vi "Graph.vi"(5 "Caption.Text":string="Frequency Responce UUT", 6 "Y Scale.Name Label.Text":string="Level/dBSPL", 7 "X Scale.Name Label.Text":string="Frequency/Hz", 9 "LimitHigh":cluster{"x-Axis":dbl[], "y-Axis":dbl[]}={"x-Axis"=[0.0, 1.0, 2.0, 3.0], "y-Axis"=[3.0, 3.0, 3.0, 3.0]}, 10 "LimitLow":cluster{"x-Axis":dbl[], "y-Axis":dbl[]}={"x-Axis"=[0.0, 1.0, 2.0, 3.0], "y-Axis"=[1.5, 1.5, 1.5, 1.5]}, 11 "Measurement":cluster{"x-Axis":dbl[], "y-Axis":dbl[]}={"x-Axis"=[0.0, 1.0, 2.0, 3.0], "y-Axis"=[1.0, 2.0, 1.5, 3.1]}) -> (0 "error out":errorcluster, 3 "output values":cluster{"frequencies":dbl[], "spectrum":dbl[]}[](graph) caption="Frequency Responce RefMicro")   [LabVIEW 2018]
uses:
  <vilib>/addons/Sound and Vibration/svt_Limit Test/SVL Limit Testing (XY).vi
  <vilib>/addons/Sound and Vibration/svt_Limit Test/SoundVib_LimitTest.lvlib
panel:
  in  "copy to clipboard":bool
  in  "stop":bool
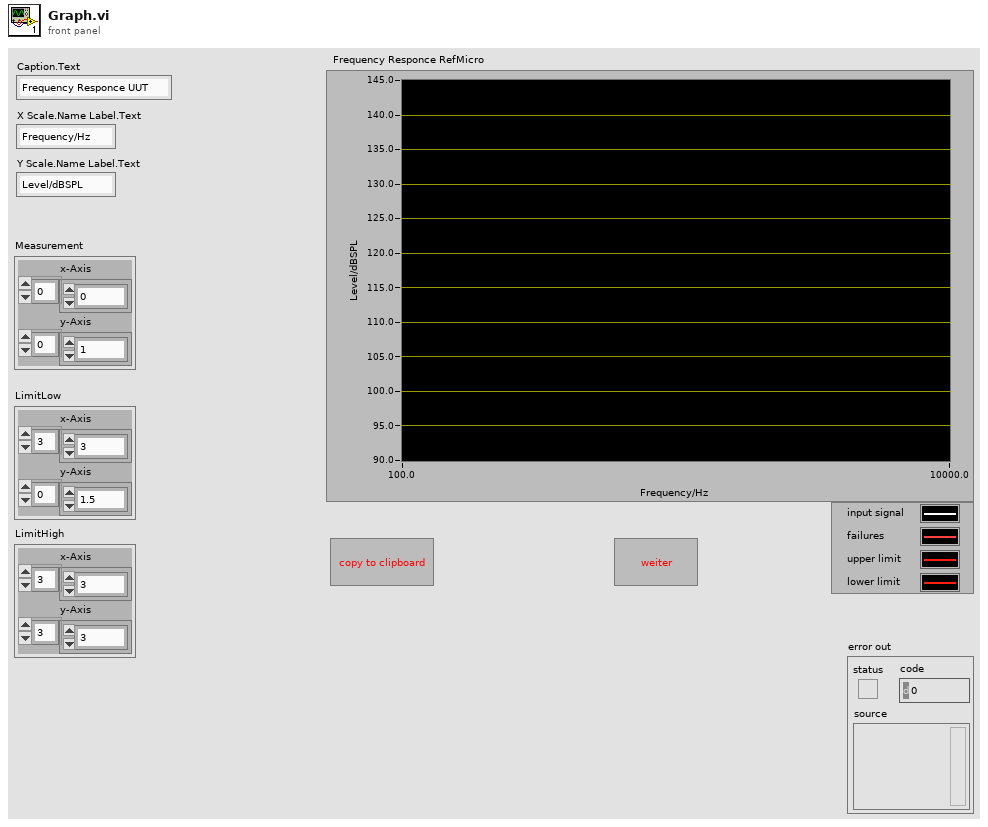
[diagram p1: front panel]
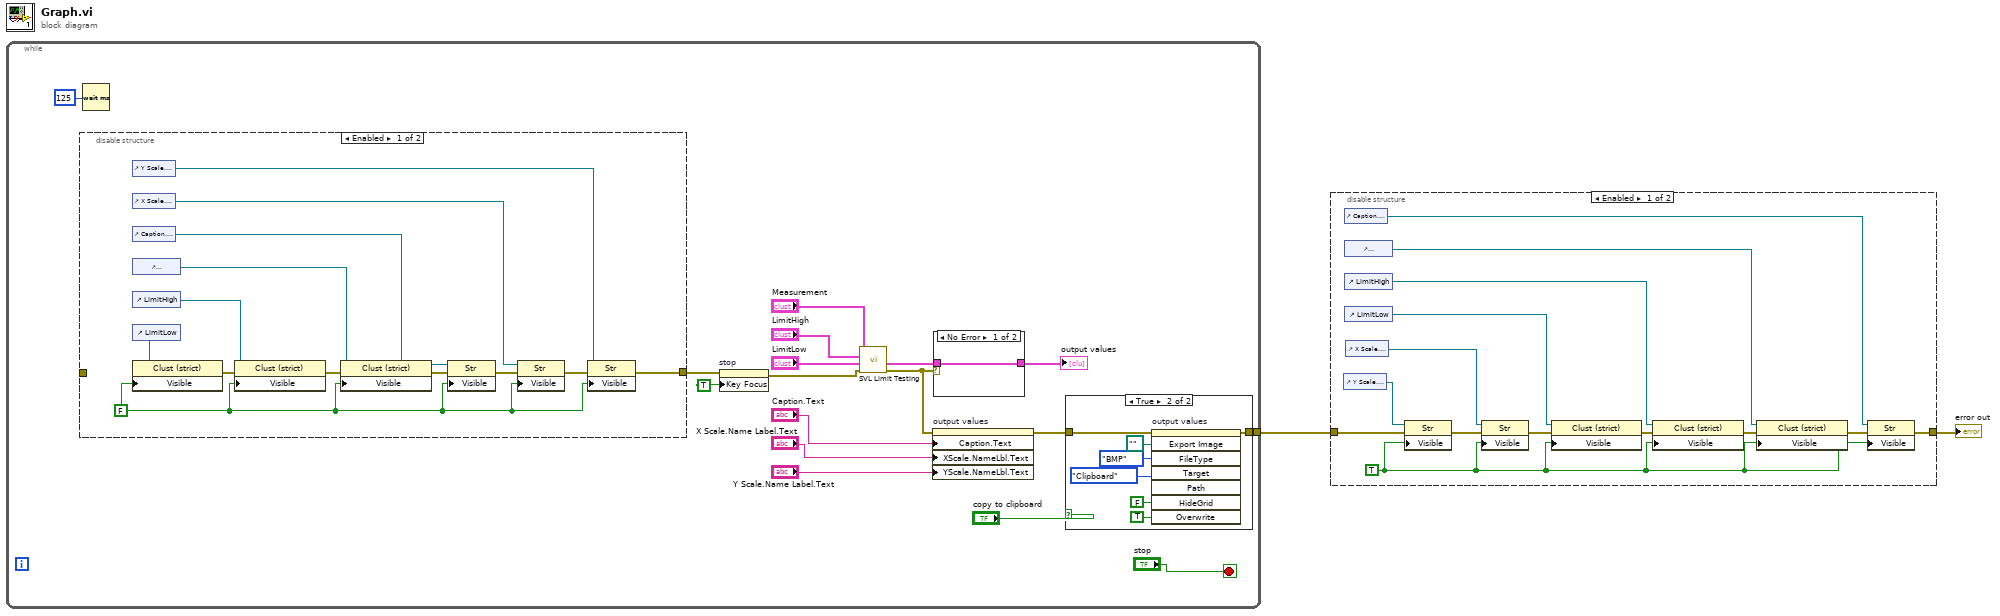
[diagram p0: block diagram]
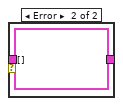
[diagram p5: hidden frame]
diagram:
  n1 = while {
    tunnel: [w7] -> w1
    stop <- "stop" stop-if-true
    n2 = disable-structure shown="Enabled" {
      disable-tunnel: [_ w41] -> _
      disable-tunnel: [w34 w41] -> w5
      frame Enabled {
        w40 = FALSE ("Visible")
        n3 = control-ref of="Y Scale.Name Label.Text"() -> (w28:refnum<vi>)
        n4 = control-ref of="X Scale.Name Label.Text"() -> (w29:refnum<vi>)
        n5 = control-ref of="Caption.Text"() -> (w30:refnum<vi>)
        n6 = control-ref of="Measurement"() -> (w31:refnum<vi>)
        n7 = control-ref of="LimitHigh"() -> (w32:refnum<vi>)
        n8 = control-ref of="LimitLow"() -> (w33:refnum<vi>)
        n9 = property on="Property Node" class="Clust (strict)"(reference=w33, "Visible"=w40) -> (error out=w39:errorcluster)  [unwired: 1 in, 1 out]
        n10 = property on="Property Node" class="Clust (strict)"(reference=w32, error in=w39, "Visible"=w40) -> (error out=w38:errorcluster)  [unwired: 1 out]
        n11 = property on="Property Node" class="Clust (strict)"(reference=w31, error in=w38, "Visible"=w40) -> (error out=w37:errorcluster)  [unwired: 1 out]
        n12 = property on="Property Node" class="Str"(reference=w30, error in=w37, "Visible"=w40) -> (error out=w36:errorcluster)  [unwired: 1 out]
        n13 = property on="Property Node" class="Str"(reference=w29, error in=w36, "Visible"=w40) -> (error out=w35:errorcluster)  [unwired: 1 out]
        n14 = property on="Property Node" class="Str"(reference=w28, error in=w35, "Visible"=w40) -> (error out=w34:errorcluster)  [unwired: 1 out]
      }
      frame Disabled {
      }
    }
    n15 = Wait (ms)(milliseconds to wait=u32 125) -> ()  [unwired: 1 out]
    n16 = property on="stop" class="Bool"(error in=w5, "Key Focus"=TRUE) -> (error out=w4:errorcluster)  [unwired: 1 in, 1 out]
    n17 = call-poly <vilib>:"SVL Limit Testing.vi"("error in (no error)"=w4, "lower limit"="LimitLow", "upper limit"="LimitHigh", "signal in"="Measurement") -> ("error out"=w14:errorcluster, "output values"=w16:cluster{"frequencies":dbl[], "spectrum":dbl[]}[])  [unwired: 4 in, 2 out]
    n18 = property on="output values" class="XYGraph (strict)"(error in=w14, "Caption.Text"="Caption.Text", "XScale.NameLbl.Text"="X Scale.Name Label.Text", "YScale.NameLbl.Text"="Y Scale.Name Label.Text") -> (error out=w8:errorcluster)  [unwired: 1 in, 1 out]
    n19 = case shown="No Error" w14 {
      tunnel: w16 -> [w42 _]
      tunnel: [w42 cluster{"frequencies":dbl[], "spectrum":dbl[]}[] [] ("output values")] -> w15
      frame No Error {
      }
      frame Error {
      }
    }
    "output values" <- w15
    n20 = case shown="True" "copy to clipboard" {
      tunnel: w8 -> [w20 w22]
      tunnel: [w20 w21] -> w7
      frame False {
      }
      frame True {
        n21 = invoke on="output values" class="XYGraph (strict)" method="Export Image"(error in=w22, "FileType"=enum32{"BMP", "EPS", "EMF", "PICT"}."BMP" ("File Type"), "Target"=enum32{"File", "Clipboard"}."Clipboard", "Path"=path "", "HideGrid"=FALSE ("Hide Grid"), "Overwrite"=TRUE ("Always Overwrite")) -> (error out=w21:errorcluster)  [unwired: 2 in, 7 out]
      }
    }
  }
  n22 = disable-structure shown="Enabled" {
    disable-tunnel: [w45 w58] -> w2
    disable-tunnel: w1 -> [w44 w58]
    frame Enabled {
      w57 = TRUE ("Visible")
      n23 = control-ref of="Y Scale.Name Label.Text"() -> (w56:refnum<vi>)
      n24 = control-ref of="Caption.Text"() -> (w47:refnum<vi>)
      n25 = control-ref of="Measurement"() -> (w46:refnum<vi>)
      n26 = control-ref of="LimitHigh"() -> (w48:refnum<vi>)
      n27 = control-ref of="LimitLow"() -> (w50:refnum<vi>)
      n28 = control-ref of="X Scale.Name Label.Text"() -> (w49:refnum<vi>)
      n29 = property on="Property Node" class="Str"(reference=w56, error in=w44, "Visible"=w57) -> (error out=w55:errorcluster)  [unwired: 1 out]
      n30 = property on="Property Node" class="Str"(reference=w49, error in=w55, "Visible"=w57) -> (error out=w54:errorcluster)  [unwired: 1 out]
      n31 = property on="Property Node" class="Clust (strict)"(reference=w50, error in=w54, "Visible"=w57) -> (error out=w53:errorcluster)  [unwired: 1 out]
      n32 = property on="Property Node" class="Clust (strict)"(reference=w48, error in=w53, "Visible"=w57) -> (error out=w52:errorcluster)  [unwired: 1 out]
      n33 = property on="Property Node" class="Clust (strict)"(reference=w46, error in=w52, "Visible"=w57) -> (error out=w51:errorcluster)  [unwired: 1 out]
      n34 = property on="Property Node" class="Str"(reference=w47, error in=w51, "Visible"=w57) -> (error out=w45:errorcluster)  [unwired: 1 out]
    }
    frame Disabled {
    }
  }
  "error out" <- w2
